vi "Horizontal Update.vi"(8 "error in (no error)":errorcluster, 10 "Horizontal Change":i16, 11 "Location":refnum<data-value>) -> (0 "error out":errorcluster, 2 "Location":T1, 3 "Location":refnum<data-value>)   [LabVIEW 2019, in "Structures.lvclass"]
uses:
  Structures.lvclass
  <vilib>/Utility/miscctls.llb/LVPointTypeDef.ctl
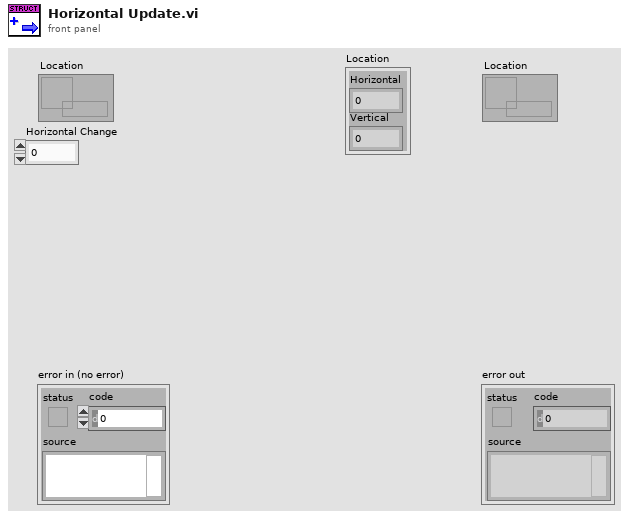
[diagram p1: front panel]
types:
  T1 = typedef "LVPointTypeDef.ctl" = cluster{"Horizontal":i16, "Vertical":i16}
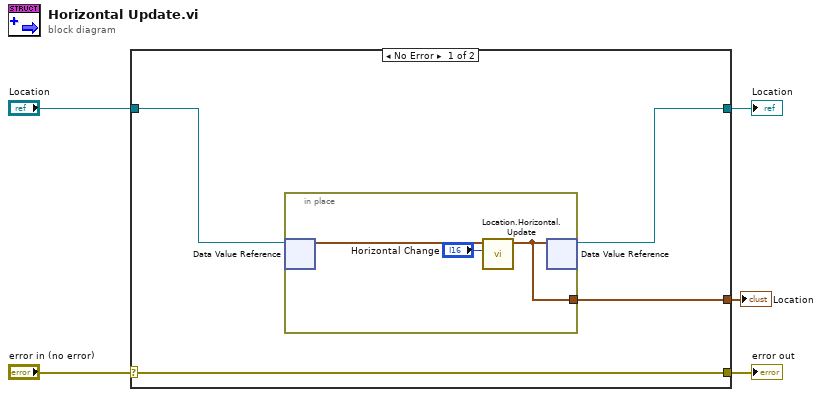
[diagram p0: block diagram]
diagram:
  n1 = case shown="No Error" "error in (no error)" {
    selector: "error in (no error)" -> [w9 w14]
    tunnel: [w9 w14] -> w4
    tunnel: [w6 w13] -> w2
    tunnel: "Location" -> [w7 w13]
    tunnel: [w8 _] -> w1
    frame No Error {
      n2 = in-place {
        in-place-border: [w10] -> w8
        n3 = in-place-dvr #1(w7) -> (w12:T1)  [unwired: 1 out]
        n4 = call "Location.Horizontal.Update.vi"("Horizontal Change"="Horizontal Change", "location in"=w12) -> ("location out"=w10:T1)  [unwired: 9 in]
        n5 = in-place-dvr #1(w10) -> (w6:refnum<data-value>)  [unwired: 1 out]
      }
    }
    frame Error {
    }
  }
  "error out" <- w4
  "Location" <- w2
  "Location" <- w1
